vi "SetTaskParameterFloat.vi"(0 "Controller In":refnum<k24>, 5 "taskId":i32(ring) items=["TLibrary", "T01", "T02", "T03", "T04", "T05", "T06", "T07", "T08", "T09", "T10", "T11", "T12", "T13", "T14", "T15", "T16", "T17", "T18", "T19", "T20", "T21", "T22", "T23", "T24", "T25", "T26", "T27", "T28", "T29", "T30", "T31"], 7 "Parameter Name":string(combo), 9 "value":sgl, 11 "error in (no error)":errorcluster) -> (4 "Controller Out":refnum<k24>, 15 "error out":errorcluster)   [LabVIEW 2010]
uses:
  c:/aerotech/controller/5.xx.xxx/A3200/pc/labview/2010/bin/Aerotech.A3200.dll
  bin/Aerotech.A3200.dll
  c:/aerotech/controller/5.xx.xxx/A3200/pc/labview/2010/bin/Aerotech.A3200.LabVIEW.dll
  bin/Aerotech.A3200.LabVIEW.dll
panel:
  out "ParameterType":i32(ring)=2 items=["Integer", "Double", "Single", "Long", "String"]
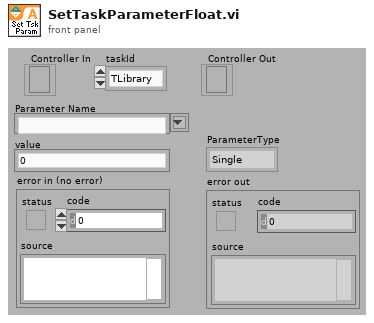
[diagram p1: front panel]
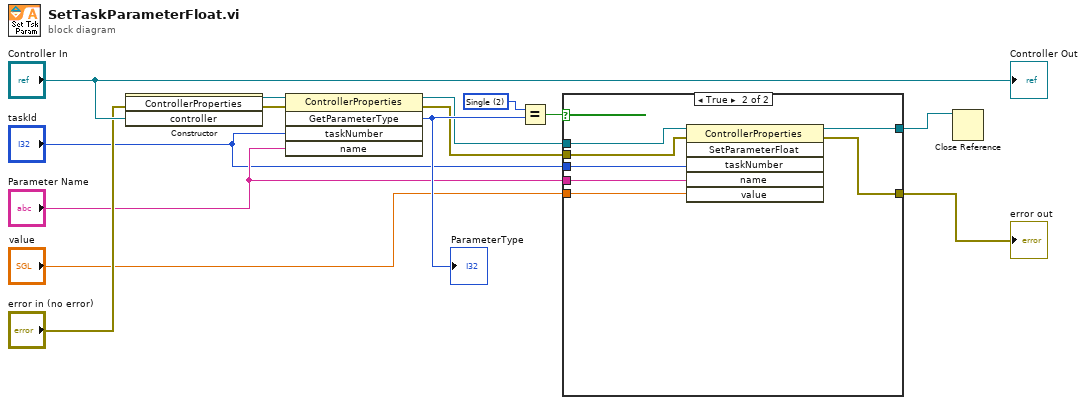
[diagram p0: block diagram]
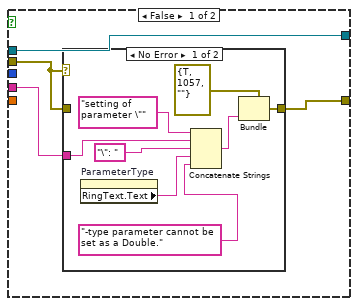
[diagram p2: hidden frame]
diagram:
  w10 = 2 items=["Integer", "Double", "Single", "Long", "String"] ("GetParameterType")
  n1 = constructor class="ControllerProperties"(error in="error in (no error)", "controller"="Controller In") -> (reference out=w12:refnum<k24>, error out=w11:errorcluster)  [unwired: 2 in, 2 out]
  n2 = invoke class="ControllerProperties" method="GetParameterType"(reference=w12, error in=w11, "taskNumber"="taskId", "name"="Parameter Name") -> (reference out=w6:refnum<k24>, error out=w5:errorcluster, "GetParameterType"=w9:i32)  [unwired: 1 in, 2 out]
  "ParameterType" <- w9
  n3 = Equal?(x=w10, y=w9) -> (x = y?=w8:bool)
  n4 = case shown="True" w8 {
    tunnel: [w18 w33] -> w7
    tunnel: w6 -> [w18 w34]
    tunnel: "Parameter Name" -> [w15 w30]
    tunnel: w5 -> [w16 w32]
    tunnel: [w17 w31] -> w4
    tunnel: "taskId" -> [_ w29]
    tunnel: "value" -> [_ w28]
    frame False {
      n5 = case shown="No Error" w16 {
        tunnel: [w25 w27] -> w17
        tunnel: w16 -> [_ w27]
        tunnel: w15 -> [w22 _]
        frame No Error {
          n6 = property on="ParameterType" class="Ring (strict)"() -> ("RingText.Text"=w20:string)  [unwired: 2 in, 2 out]
          n7 = Concatenate Strings("setting of parameter \"" ("string"), w22, "\": " ("string"), w20, "-type parameter cannot be set as a Double." ("string")) -> (w24:string)
          n8 = Bundle(cluster=cluster{bool, "code":i32, "source":string} {TRUE, "code"=1057, "source"=""} ("error out"), "source"=w24) -> (w25:cluster{bool, "code":i32, "source":string})  [unwired: 2 in]
        }
        frame Error {
        }
      }
    }
    frame True {
      n9 = invoke class="ControllerProperties" method="SetParameterFloat"(reference=w34, error in=w32, "taskNumber"=w29, "name"=w30, "value"=w28) -> (reference out=w33:refnum<k24>, error out=w31:errorcluster)  [unwired: 1 in, 4 out]
    }
  }
  "error out" <- w4
  n10 = Close Reference(reference=w7) -> ()  [unwired: 1 in, 1 out]
  "Controller Out" <- "Controller In"
